vi "flushTank.vi"(8 "error in (no error)":errorcluster, 10 "Index":i32, 11 "Tank in":refnum<class "Tank.lvclass">) -> (0 "error out":errorcluster, 3 "Tank out":refnum<class "Tank.lvclass">)   [LabVIEW 2017, in "Tank.lvclass"]
uses:
  Tank.lvclass
  Tank.lvclass/Tank.ctl
  Sensor Class/Sensor.lvclass/Sensor.ctl
  Sensor Class/Sensor.lvclass
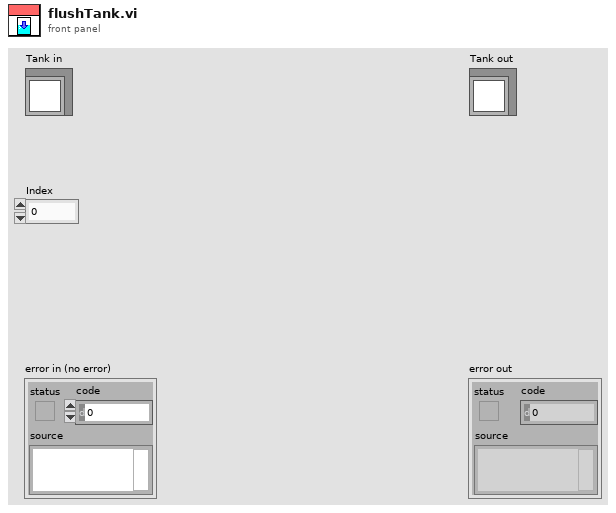
[diagram p1: front panel]
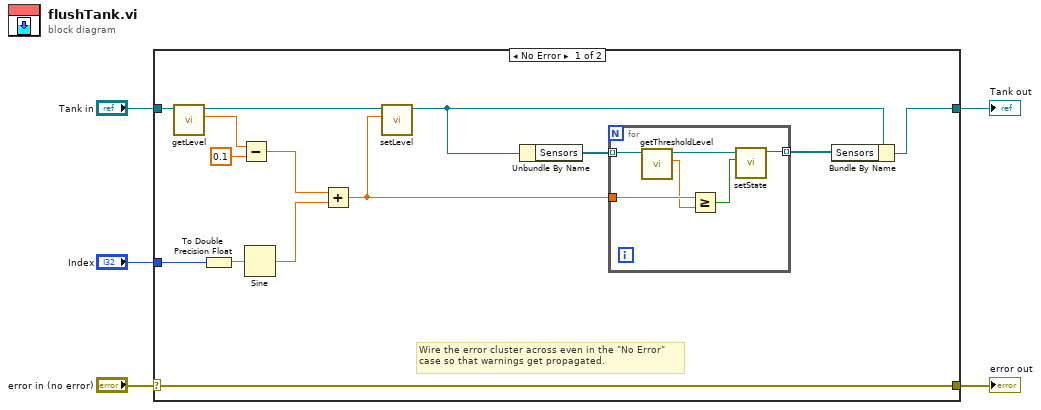
[diagram p0: block diagram]
diagram:
  n1 = case shown="No Error" "error in (no error)" {
    selector: "error in (no error)" -> [w19 w27]
    tunnel: [w19 w27] -> w4
    tunnel: [w17 w26] -> w2
    tunnel: "Tank in" -> [w18 w26]
    tunnel: "Index" -> [w12 _]
    frame No Error {
      # "Wire the error cluster across even in the \"No Error\"\ncase so that warnings get propagated."
      n2 = call "getLevel.vi"("Tank in"=w18) -> ("Level"=w11:dbl, "Tank out"=w9:refnum<class "Tank.lvclass">)  [unwired: 8 in, 1 out]
      n3 = To Double Precision Float(number=w12) -> (double precision float=w16:dbl)
      n4 = Subtract(x=w11, y=0.1 ("x")) -> (x-y=w14:dbl)
      n5 = Sine(x=w16) -> (sin(x)=w15:dbl)
      n6 = Add(x=w14, y=w15) -> (x+y=w6:dbl)
      n7 = call "setLevel.vi"("Level"=w6, "Tank in"=w9) -> ("Tank out"=w8:refnum<class "Tank.lvclass">)  [unwired: 8 in, 1 out]
      n8 = Unbundle By Name(w8) -> ("Sensors"=w10:refnum<class "Sensor.lvclass">[])
      n9 = for {
        tunnel: w10 -> [w25] mode=indexing
        tunnel: w6 -> [w21]
        tunnel: [w22] -> w7 mode=indexing
        n10 = call "getThresholdLevel.vi"("Sensor in"=w25) -> ("Threshold Level"=w20:dbl, "Sensor out"=w24:refnum<class "Sensor.lvclass">)  [unwired: 8 in, 1 out]
        n11 = Greater Or Equal?(x=w21, y=w20) -> (x >= y?=w23:bool)
        n12 = call "setState.vi"("State"=w23, "Sensor in"=w24) -> ("Sensor out"=w22:refnum<class "Sensor.lvclass">)  [unwired: 8 in, 1 out]
      }
      n13 = Bundle By Name(cluster=w8, "Sensors"=w7) -> (w17:refnum<class "Tank.lvclass">)
    }
    frame Error {
    }
  }
  "error out" <- w4
  "Tank out" <- w2
